vi "Agilent 34970 HEWH Example Scan.vi"() -> ()   [LabVIEW 2020]
uses:
  Trunk/Utility/Save File/File Setup (Public)/Type Definition/Save File DOE LabView Program.ctl
  Agilent 34970.lvlib
  Trunk/Utility/Save File/File Setup.lvlib
panel:
  in  "LV Program":T1=enum."Gas Water Heater"
  in  "stop":bool
  out "Output Array":dbl[](array[numeric]) format="%.2f"
  in  "VISA Resource Name":refnum<visa-resource-name>
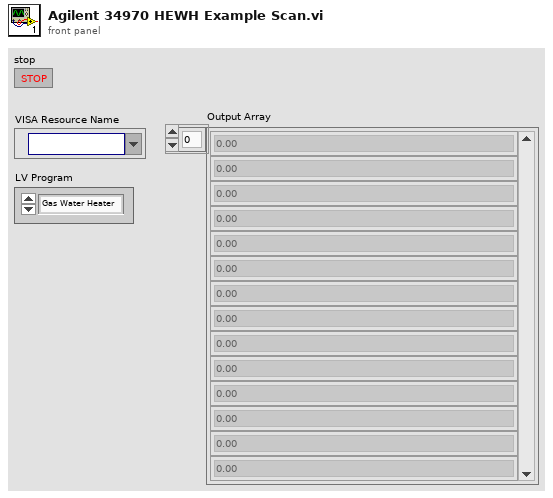
[diagram p1: front panel]
types:
  T1 = typedef "File Setup.lvlib/Save File DOE LabView Program.ctl" = enum16{"No Name Found", "DOE Stand", "Dishwasher Kitchen", "Portable Stand", "HEWH", "Dryer", "Dryer WILT", "HCC", "PRAT", "HEWH RLT", "Refrigeration", "Gas Water Heater"}
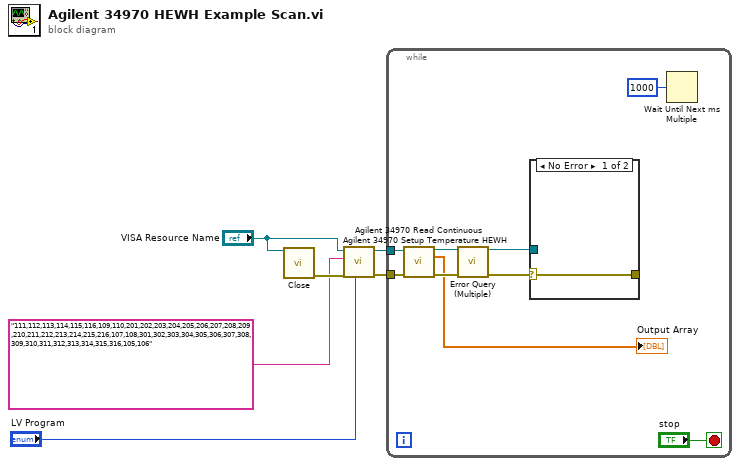
[diagram p0: block diagram]
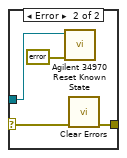
[diagram p2: hidden frame]
diagram:
  n1 = call "Close.vi"("VISA Resource Name"="VISA Resource Name") -> ("error out"=w6:errorcluster)  [unwired: 14 in]
  n2 = call "Agilent 34970 Setup Temperature HEWH.vi"("LV Program"="LV Program", "Error In"=w6, "Agilent Channel Input"="111,112,113,114,115,116,109,110,201,202,203,204,205,206,207,208,209,210,211,212,213,214,215,216,107,108,301,302,303,304,305,306,307,308,309,310,311,312,313,314,315,316,105,106", "VISA Refnum in"="VISA Resource Name") -> ("Error Out"=w2:errorcluster, "VISA Resource Name Out"=w3:refnum<visa-resource-name>)  [unwired: 6 in]
  n3 = while {
    tunnel: w3 -> [w13]
    tunnel: w2 -> [w12]
    stop <- "stop" stop-if-true
    n4 = call "Agilent 34970 Read Continuous.vi"("VISA Resource Name"=w13, "error in (no error)"=w12) -> ("VISA resource name out"=w15:refnum<visa-resource-name>, "Output Array"=→"Output Array":dbl[], "error out"=w14:errorcluster)  [unwired: 10 in, 1 out]
    n5 = call "Error Query (Multiple).vi"("VISA Resource Name"=w15, "error in (no error)"=w14) -> ("VISA Resource Name Out"=w10:refnum<visa-resource-name>, "error out"=w11:errorcluster)  [unwired: 10 in, 2 out]
    n6 = case shown="No Error" w11 {
      selector: w11 -> [w16 w18]
      tunnel: [w16 w17] -> _
      tunnel: w10 -> [_ w20]
      frame No Error {
      }
      frame Error {
        n7 = call "Agilent 34970 Reset Known State.vi"("Error In"=errorcluster {"status"=TRUE, "code"=0, "source"=""}, "VISA Refnum in"=w20) -> ()  [unwired: 9 in, 1 out]
        n8 = call <vilib>:"Clear Errors.vi"("error in (no error)"=w18) -> ("error out"=w17:errorcluster)  [unwired: 5 in, 1 out]
      }
    }
    n9 = Wait Until Next ms Multiple(millisecond multiple=u32 1000) -> ()  [unwired: 1 out]
  }
